vi "TimerEngine.WaitforEngineStarted.vi"(8 "error in (no error)":errorcluster, 11 "DVR":refnum<data-value>) -> (0 "error out":errorcluster, 3 "DVR 2":refnum<data-value>)   [LabVIEW 2017, in "TimerEngine.lvlib" / "TimerEngine.lvclass"]
uses:
  TimerEngine.lvclass
  TimerEngine.lvclass/TimerEngine.ctl
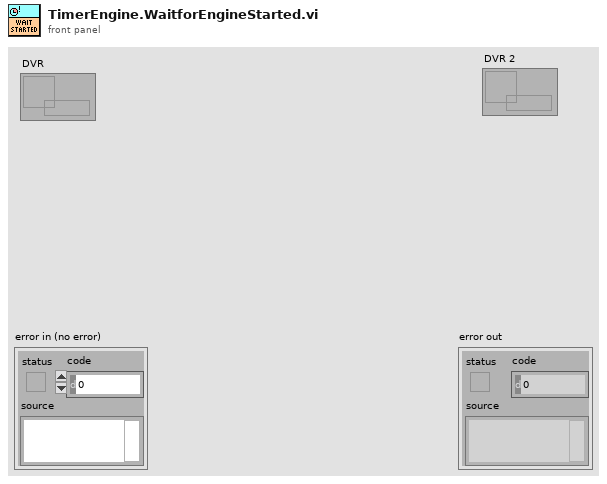
[diagram p1: front panel]
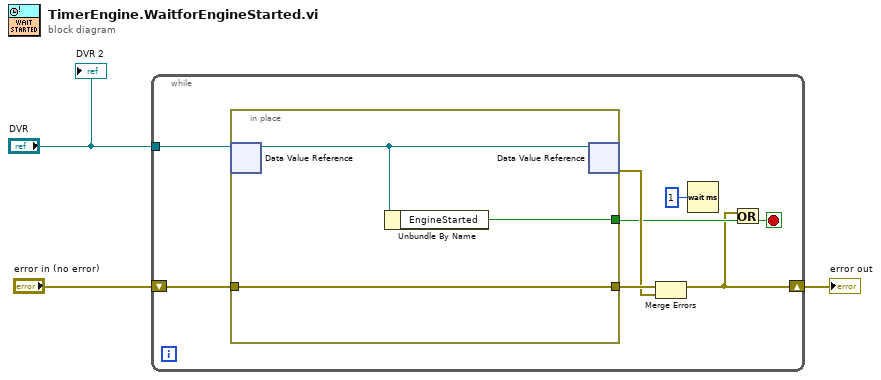
[diagram p0: block diagram]
diagram:
  n1 = while {
    tunnel: "DVR" -> [w11]
    shift-right: [w5] -> w2
    shift-left: "error in (no error)" -> [w9]
    stop <- w6 stop-if-true
    n2 = in-place {
      in-place-border: [w14] -> w10
      in-place-border: w9 -> [w14]
      in-place-border: [w12] -> w7
      n3 = in-place-dvr #1(w11) -> (w13:refnum<class "TimerEngine.lvclass">)  [unwired: 1 out]
      n4 = Unbundle By Name(w13) -> ("EngineStarted"=w12:bool)
      n5 = in-place-dvr #1(w13) -> (w8:errorcluster)  [unwired: 1 out]
    }
    n6 = Merge Errors(w10, w8) -> (w5:errorcluster)
    n7 = Wait (ms)(milliseconds to wait=u32 1) -> ()  [unwired: 1 out]
    n8 = Or(x=w5, y=w7) -> (x .or. y?=w6:bool)
  }
  "error out" <- w2
  "DVR 2" <- "DVR"
